vi "event.create.vi"(6 "Type":enum16{"INFO", "FLAG", "ERROR", "SUCCESS"}(ring), 7 "Time Stamp (now: system time)":timestamp format="%<%x %.3X>T", 8 "error in":errorcluster, 9 "Name":string, 10 "assets":refnum<class "asset.lvclass">[](array[class]), 11 "Nominal Client in":refnum<class "Nominal Client.lvclass">) -> (0 "error out":errorcluster, 2 "event":refnum<class "event.lvclass">, 3 "Nominal Client out":refnum<class "Nominal Client.lvclass">)   [LabVIEW 2020, in "Nominal Client.lvclass"]
doc: "Creates a timestamped event in Nominal associated with one or more assets, marking significant occurrences during test execution such as hardware state changes or sequence transitions. Events appear alongside telemetry data to enable correlation between test activities and system behavior during analysis."
uses:
  Nominal Client.lvclass
  Nominal Client.lvclass/Nominal Client.ctl
  event/event.lvclass
  asset/asset.lvclass
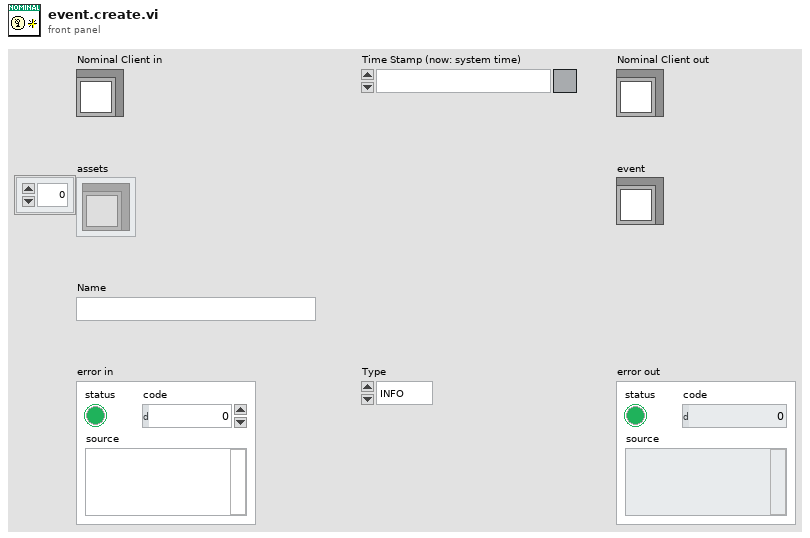
[diagram p1: front panel]
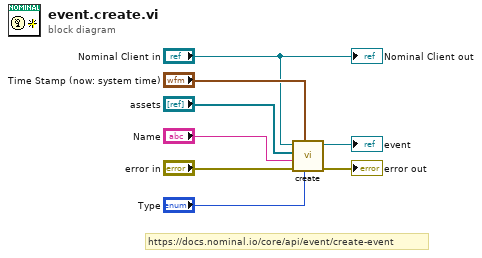
[diagram p0: block diagram]
diagram:
  # "https://docs.nominal.io/core/api/event/create-event"
  n1 = call "create.vi"("Type"="Type", "Time Stamp (now)"="Time Stamp (now: system time)", "error in"="error in", "Name"="Name", "assets"="assets", "Nominal Client in"="Nominal Client in") -> ("error out"=→"error out":errorcluster, "event"=→"event":refnum<class "event.lvclass">)  [unwired: 4 in]
  "Nominal Client out" <- "Nominal Client in"
